vi "test-ramsete-path.vi"() -> ()   [LabVIEW 2019]
uses:
  Pathfinder-Lib/VIs/Waypoint.ctl
  Pathfinder-Lib/VIs/Wheel_Ctrl_Path_Element.ctl
  PathExecution_Library/PATH_SAMPLE.ctl
  PathExecution_Library/POSE.ctl
  PathExecution_Library/TRANSLATION.ctl
  PathExecution_Library/ROTATION.ctl
  Pathfinder-Lib/VIs/Wheel_Ctrl_Path.ctl
  Pathfinder-Lib/Pathfinder.lvlib
  Secret_Control_Library_Protected/Secret_Control_Library_Protected.lvlib
  PathExecution_Library/PathExecution_Library.lvlib
panel:
  in  "Tab Control 3":enum32{"Robot Data", "Path Definition"}(tab)
  in  "Real max\n speed":dbl=96.0
  in  "wheelbase_width":dbl=20.866
  in  "max_jerk":dbl=90.0
  in  "max_acceleration":dbl=65.0
  in  "max_velocity":dbl=72.0
  in  "?":T1[](array[typedef])=[{"x"=15.0, "y"=105.0, "angle"=0.0}, {"x"=35.0, "y"=105.0, "angle"=0.0}, {"x"=210.0, "y"=185.0, "angle"=60.0}]
  in  "Path Results\ndT":dbl=0.02 format="%7.3f"
  in  "sample_count":i32=100000
  out "Path calculation error":errorcluster
  in  "Calculate\nPath":bool
  out "Complete,\nReady to \nExecute":bool
  out "Path \nSpeed > \nMax":bool
  in  "Rev\nDirection":bool
  out "max speed":dbl
  in  "Tab Control 2":T2(tab)
  in  "Enable Ramsete":bool=TRUE
  out "Distance":dbl[](array[numeric]) format="%19.2f"
  in  "Execute\nRobot":bool
  out "Robot\nExecuting":bool
  in  "Stop\nProgram":bool
  out "Speed":dbl[](array[numeric]) format="%19.2f"
  out "SpeedDmd":dbl[](array[numeric]) format="%19.2f"
  in  "Next Step":bool
  in  "Include Step":bool=TRUE
  in  "End Path CMD":i32=64
  in  "Cont Path CMD":i32=62
  in  "Start Path CMD":i32=60
  in  "Starting Step":i32
  in  "Command List Path Comment":string
  in  "Command List File Name":path
  in  "CreateCmdList":bool
  in  "CreateCmdList 2":bool
  in  "Command List File Name 2":path
  in  "Command List Path Comment 2":string
  in  "Starting Step 2":i32
  in  "Start Path CMD 2":i32=80
  in  "Cont Path CMD 2":i32=82
  in  "End Path CMD 2":i32=84
  in  "Include Step 2":bool=TRUE
  in  "Tab Control":T3(tab)
  out "Position":cluster{dbl[], dbl[]}[](graph)
  out "Path":T4(graph)
  out "Size":i32
  out "Robot Path Data":T5[](array[typedef]) {"D Time" format="%13.3f"; "Angle" format="%13.3f"; "R dist" format="%13.3f"; "L dist" format="%13.3f"; "R spd" format="%13.3f"; "L spd" format="%13.3f"; "T Time" format="%13.3f"}
  out "Ramsete Path":T6[](array[typedef])
  out "element":T6
  out "AtReference":bool
  out "size(s)":i32
  out "Path INX":i32
  out "size(s) 2":i32
  out "Err Pose":T7 {"ROTATION"."SIN" format="%10.3f"; "ROTATION"."COS" format="%10.3f"; "ROTATION"."VALUE" format="%10.3f"; "TRANSLATION"."Y" format="%9.3f"; "TRANSLATION"."X" format="%10.3f"}
  out "CurrentRelativePose":T7
  out "Des Pose":T7
  # "ROBOT DATA"
  # "INCHES/SEC"
  # "INCHES/SEC"
  # "INCHES/SEC^2"
  # "?? INCHES/SEC^3"
  # "Simulated robot is 20.866"
  # "INCHES"
  # "PATH DEFINITION"
  # "SEC"
  # "ROBOT EXECUTION"
  # "Instructions:\nThis should create a path, show the data on the various tabs and optionally write the motor demands and expected results to a file for use on a a robot..\n1) Enter robot data on Robot Data Tab\n2) Define your path definitions.\n3) Define the time increment.  0.020 is chosen since that matches the normal loop time.\n4) Press calculate path.  If a good path was calculated it will be displayed on the Tank Data tab, and the Ready to Execute will indicate execution can begin.\nThe path can be recalculated many times before selecting execute.\n\nTo write to a file.\n5) Select the file name\n6) This example uses \"steps\", sequential numbers for inclusion into a list based autonomous routine.  Including the step number if optional.\n7) This uses command numbers to indicate first, last, and intermediate steps.  This allows some simplification of the execution routine.  It\nalso allows the path to be executed backwards if desired.  The command numbers are changeable.\n8) Press \"Create Command List\".\n\nNotes:\n- PC robot simulataion is disabled in this program.  The code is still there if you want to restore it and try it out.  Use one of the other test programs \nto simulate the path on a PC.\n- The path generation logic doesn't account distribution of speed to the left and right wheels.  As a result the maximum speed can be exceeded.\nIf this happens, but Path Speed > Max light will light and Ready to Execute will not light.  Lower the maximum speed in the Robot Data tab\nand recalulate the path.\n- 2019 playing field size - width: 26 ft 11.25 In = 323.25 in , length: 52 ft 5.25 in = 629.25 in  (I didn't verify this for the 2020 version.)"
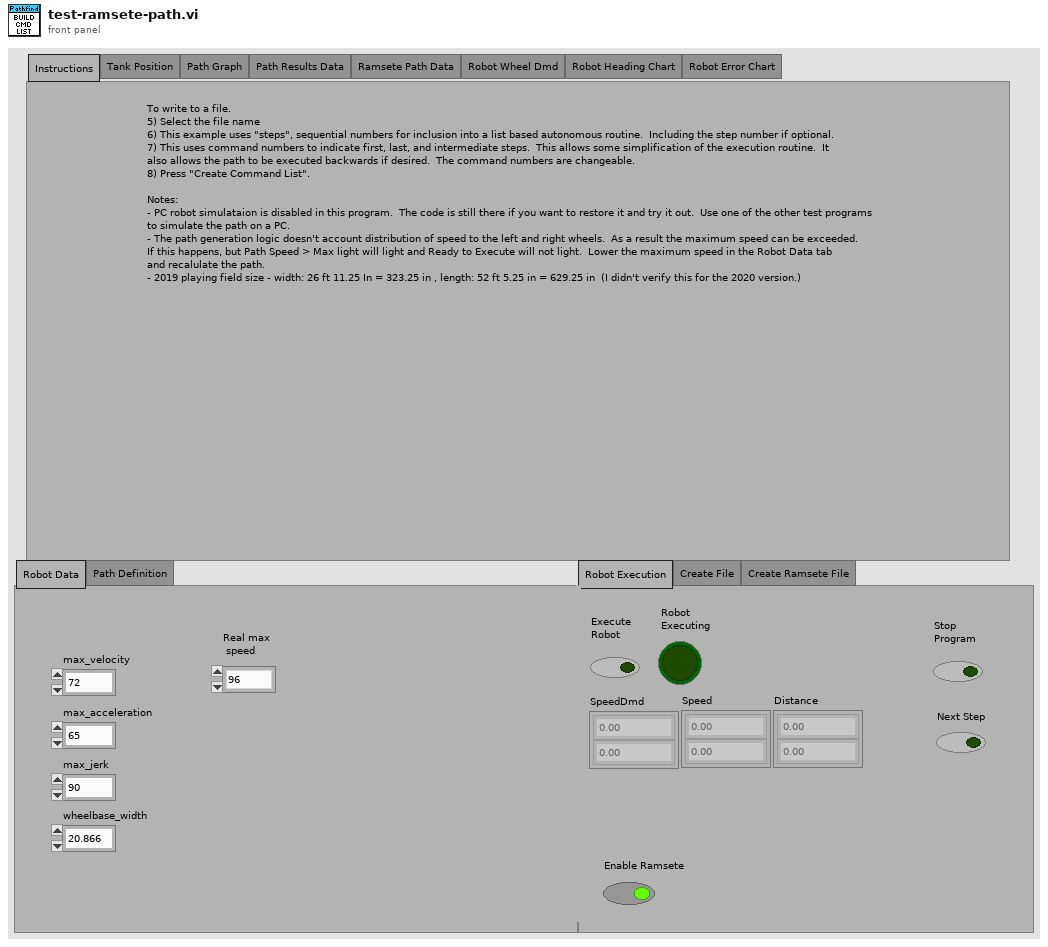
[diagram p1: front panel]
types:
  T1 = typedef "Pathfinder.lvlib/Waypoint.ctl" = cluster{"x":dbl, "y":dbl, "angle":dbl}
  T2 = enum32{"Robot Execution", "Create File", "Create Ramsete File"}
  T3 = enum32{"Instructions", "Tank Position", "Path Graph", "Path Results Data", "Ramsete Path Data", "Robot Wheel Dmd", "Robot Heading Chart", "Robot Error Chart"}
  T4 = cluster{"position":dbl, "velocity":dbl, "acceleration":dbl, "jerk":dbl, "heading":dbl}[]
  T5 = typedef "Pathfinder.lvlib/Wheel_Ctrl_Path_Element.ctl" = cluster{"T Time":dbl, "L spd":dbl, "R spd":dbl, "L dist":dbl, "R dist":dbl, "Angle":dbl, "D Time":dbl}
  T6 = typedef "PathExecution_Library.lvlib/PATH_SAMPLE.ctl" = cluster{"Path Lin Vel":dbl, "Path Ang Vel":dbl, "Path X":dbl, "Path Y":dbl, "Path Heading":dbl, "Path Time Off":dbl}
  T7 = typedef "PathExecution_Library.lvlib/POSE.ctl" = cluster{"TRANSLATION":T8, "ROTATION":T9}
  T8 = typedef "PathExecution_Library.lvlib/TRANSLATION.ctl" = cluster{"X":dbl, "Y":dbl}
  T9 = typedef "PathExecution_Library.lvlib/ROTATION.ctl" = cluster{"VALUE":dbl, "COS":dbl, "SIN":dbl}
  T10 = typedef "Pathfinder.lvlib/Wheel_Ctrl_Path.ctl" = cluster{"Wheel_Ctrl_Elements":T5[], "NumberOfElements":u32, "DeltaMillseconds":i32}
  T11 = typedef "Pathfinder.lvlib/Segment.ctl" = cluster{"dt":dbl, "x":dbl, "y":dbl, "position":dbl, "velocity":dbl, "acceleration":dbl, "jerk":dbl, "heading":dbl}
  T12 = cluster{"position":dbl, "velocity":dbl, "acceleration":dbl, "jerk":dbl, "heading":dbl}
  T13 = typedef "PathExecution_Library.lvlib/CHASSIS.ctl" = cluster{"vX":dbl, "vY":dbl, "vOmega":dbl}
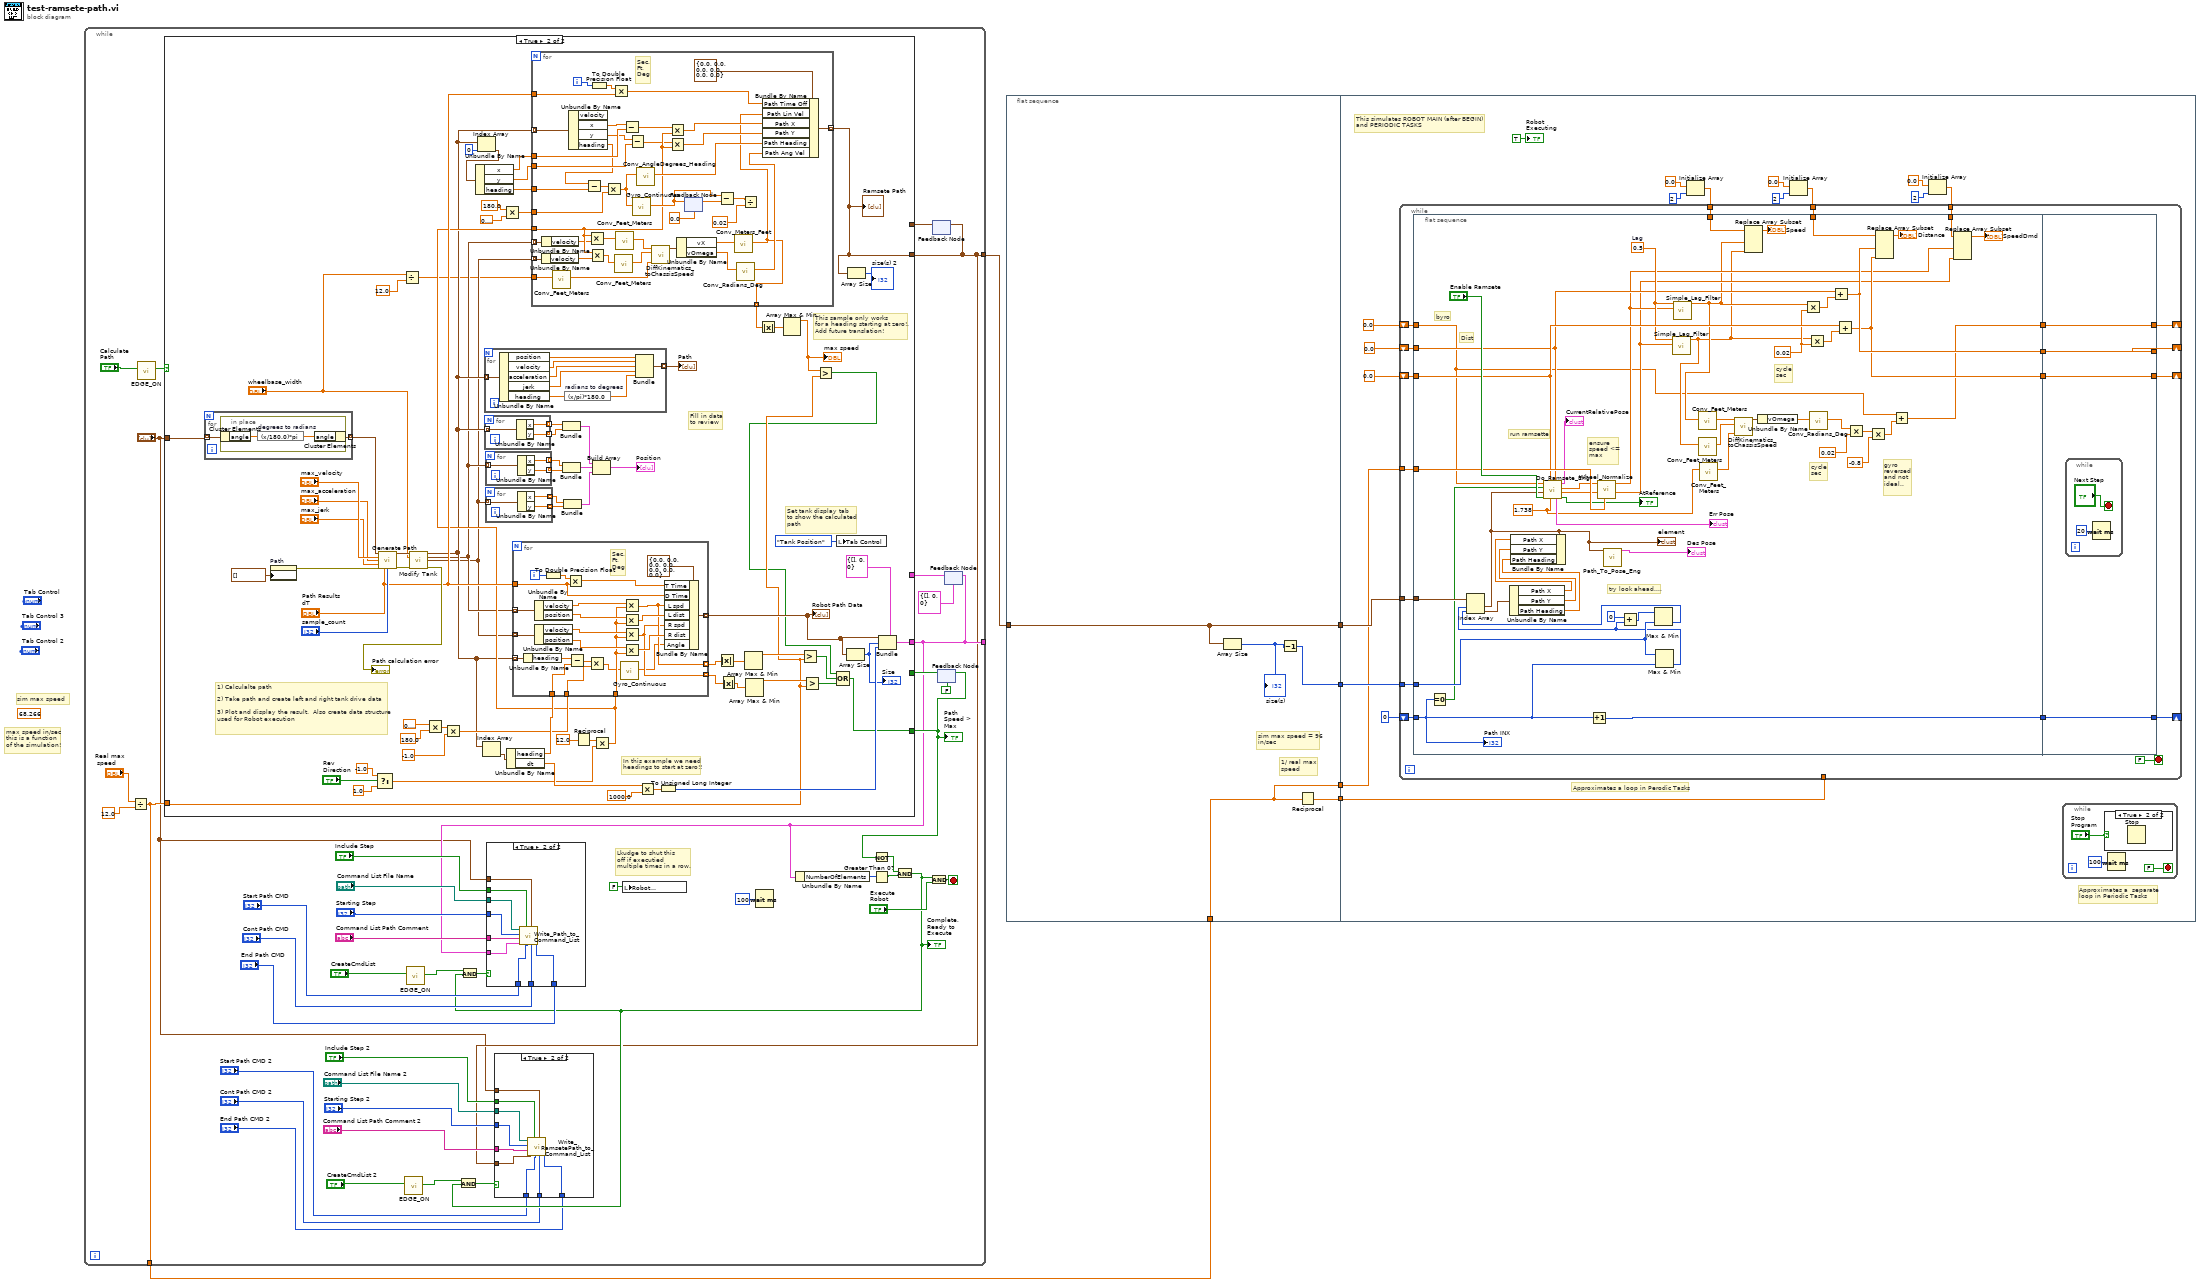
[diagram p0: block diagram]
diagram:
  (unwired) 68.266 ("x")
  # "sim max speed"
  # "max speed in/sec\nthis is a function\nof the simulation!"
  n1 = while {
    tunnel: [w22] -> w6
    tunnel: [w21] -> _
    tunnel: [w8] -> w4
    stop <- w41 stop-if-true
    # "Lkudge to shut this\noff if executied\nmultiple times in a row."
    n2 = Divide(x="Real max\n speed", y=12.0) -> (x/y=w22:dbl)
    n3 = call "EDGE_ON.vi"("INPUT"="Calculate\nPath") -> ("EDGE ON"=w46:bool)  [unwired: 10 in]
    n4 = call "EDGE_ON.vi"("INPUT"="CreateCmdList 2") -> ("EDGE ON"=w15:bool)  [unwired: 10 in]
    n5 = call "EDGE_ON.vi"("INPUT"="CreateCmdList") -> ("EDGE ON"=w29:bool)  [unwired: 10 in]
    n6 = local write "Robot\nExecuting"(FALSE ("Robot\nExecuting")) -> ()
    n7 = Wait (ms)(milliseconds to wait=u32 100) -> ()  [unwired: 1 out]
    n8 = feedback #1() -> (w20:T6[])  [unwired: 1 in]
    n9 = feedback #2(FALSE) -> (w38:bool)
    n10 = feedback #3(T10 {"Wheel_Ctrl_Elements"=[], "NumberOfElements"=0, "DeltaMillseconds"=0} ("Wheel_Ctrl_Elements")) -> (w44:T10)
    n11 = case shown="True" w46 {
      tunnel: [w69 w113] -> w21
      tunnel: w44 -> [w69 _]
      tunnel: w22 -> [_ w72]
      tunnel: [w68 w110] -> w35
      tunnel: w38 -> [w68 _]
      tunnel: "?" -> [_ w108]
      tunnel: [w67 w92] -> w8
      tunnel: w20 -> [w67 _]
      frame False {
      }
      frame True {
        # "This sample only works\nfor a heading starting at zero!.\nAdd future translation!"
        # "Set tank display tab\nto show the calculated\npath"
        # "Fill in data\nto review"
        # "1) Calculalte path\n\n2) Take path and create left and right tank drive data\n\n3) Plot and display the result.  Also create data structure\nused for Robot execution"
        # "In this example we need\nheadings to start at zero!!"
        n12 = for {
          tunnel: w108 -> [w213] mode=indexing
          tunnel: [w212] -> w138 mode=indexing
          n13 = in-place {
            n14 = in-place-cluster #4(w213) -> ("angle"=w215:dbl)
            n15 = expression code="(x/180.0)*pi" "degrees to radians"(w215) -> (w214:dbl)
            n16 = in-place-cluster #4("angle"=w214) -> (w212:T1)
          }
        }
        n17 = property on="Path" class="WFChart (strict)"("History Data"=T4 []) -> (error out=w139:errorcluster)  [unwired: 2 in, 1 out]
        n18 = Select(t=-1.0, s="Rev\nDirection", f=1.0) -> (s? t:f=w103:dbl)
        n19 = call "Generate Path.vi"("path"=w138, "max_velocity"="max_velocity", "max_acceleration"="max_acceleration", "max_jerk"="max_jerk", "error in"=w139, "dt (.001)"="Path Results\ndT", "sample_count (100000)"="sample_count") -> ("Segments"=w140:T11[], "error out"=w128:errorcluster)  [unwired: 7 in]
        n20 = Divide(x="wheelbase_width", y=12.0) -> (x/y=w82:dbl)
        n21 = call "Modify Tank.vi"("Original"=w140, "wheelbase_width"="wheelbase_width", "error in"=w128) -> ("original"=w97:T11[], "left"=w86:T11[], "right"=w85:T11[], "error out"=→"Path calculation error":errorcluster)  [unwired: 9 in]
        n22 = Multiply(x=0.3183098861837907, y=180.0) -> (x*y=w144:dbl)
        n23 = Multiply(x=w144, y=-1.0) -> (x*y=w100:dbl)
        n24 = Index Array(array=w97, index=0) -> (element=w95:T11)
        n25 = Unbundle By Name(w95) -> ("x"=w94:dbl, "y"=w93:dbl, "heading"=w90:dbl)
        n26 = Index Array(array=w97) -> (element=w145:T11)  [unwired: 1 in]
        n27 = for {
          tunnel: w97 -> [w232] mode=indexing
          tunnel: [w226] -> w142 mode=indexing
          n28 = Unbundle By Name(w232) -> ("position"=w231:dbl, "velocity"=w230:dbl, "acceleration"=w229:dbl, "jerk"=w228:dbl, "heading"=w227:dbl)
          n29 = expression code="(x/pi)*180.0" "radians to degrees"(w227) -> (w225:dbl)
          n30 = Bundle("position"=w231, "velocity"=w230, "acceleration"=w229, "jerk"=w228, "heading"=w225) -> (w226:T12)  [unwired: 1 in]
        }
        "Path" <- w142
        n31 = for {
          tunnel: w97 -> [w218] mode=indexing
          tunnel: [w217] -> w135 mode=indexing
          tunnel: [w216] -> w136 mode=indexing
          n32 = Unbundle By Name(w218) -> ("x"=w217:dbl, "y"=w216:dbl)
        }
        n33 = for {
          tunnel: w86 -> [w224] mode=indexing
          tunnel: [w223] -> w129 mode=indexing
          tunnel: [w222] -> w130 mode=indexing
          n34 = Unbundle By Name(w224) -> ("x"=w223:dbl, "y"=w222:dbl)
        }
        n35 = for {
          tunnel: w85 -> [w221] mode=indexing
          tunnel: [w220] -> w131 mode=indexing
          tunnel: [w219] -> w132 mode=indexing
          n36 = Unbundle By Name(w221) -> ("x"=w220:dbl, "y"=w219:dbl)
        }
        n37 = Multiply(x=180.0, y=0.3183098861837907) -> (x*y=w87:dbl)
        n38 = Unbundle By Name(w145) -> ("heading"=w101:dbl, "dt"=w117:dbl)
        n39 = Bundle(w135, w136) -> (w137:cluster{dbl[], dbl[]})  [unwired: 1 in]
        n40 = Bundle(w129, w130) -> (w134:cluster{dbl[], dbl[]})  [unwired: 1 in]
        n41 = Bundle(w131, w132) -> (w133:cluster{dbl[], dbl[]})  [unwired: 1 in]
        n42 = Reciprocal(x=12.0) -> (1/x=w107:dbl)
        n43 = Build Array(w137, w134, w133) -> (→"Position":cluster{dbl[], dbl[]}[])
        n44 = Multiply(x=w107, y=w103) -> (x*y=w99:dbl)
        n45 = for {
          tunnel: "Path Results\ndT" -> [w207]
          tunnel: [w210] -> w109 mode=indexing
          tunnel: w99 -> [w202]
          tunnel: w86 -> [w199] mode=indexing
          tunnel: w85 -> [w198] mode=indexing
          tunnel: w97 -> [w197] mode=indexing
          tunnel: w101 -> [w190]
          tunnel: [w193] -> w81 mode=indexing
          tunnel: [w192] -> w78 mode=indexing
          tunnel: w100 -> [w191]
          i -> [w209]
          # "Sec,\nFt,\nDeg"
          n46 = Unbundle By Name(w197) -> ("heading"=w195:dbl)
          n47 = Unbundle By Name(w199) -> ("velocity"=w206:dbl, "position"=w205:dbl)
          n48 = Unbundle By Name(w198) -> ("velocity"=w204:dbl, "position"=w203:dbl)
          n49 = To Double Precision Float(number=w209) -> (double precision float=w211:dbl)
          n50 = Multiply(x=w211, y=w207) -> (x*y=w208:dbl)
          n51 = Subtract(x=w195, y=w190) -> (x-y=w196:dbl)
          n52 = Multiply(x=w196, y=w191) -> (x*y=w189:dbl)
          n53 = call "Gyro_Continuous.vi"("GyroInput"=w189) -> ("GyroContinuous"=w188:dbl)  [unwired: 10 in]
          n54 = Multiply(x=w206, y=w202) -> (x*y=w193:dbl)
          n55 = Multiply(x=w205, y=w202) -> (x*y=w201:dbl)
          n56 = Multiply(x=w204, y=w202) -> (x*y=w192:dbl)
          n57 = Multiply(x=w203, y=w202) -> (x*y=w200:dbl)
          n58 = Bundle By Name(cluster=T5 {"T Time"=0.0, "L spd"=0.0, "R spd"=0.0, "L dist"=0.0, "R dist"=0.0, "Angle"=0.0, "D Time"=0.0} ("Wheel dmd"), "T Time"=w208, "D Time"=w207, "L spd"=w193, "L dist"=w201, "R spd"=w192, "R dist"=w200, "Angle"=w188) -> (w210:T5)
        }
        "Robot Path Data" <- w109
        n59 = for {
          tunnel: "Path Results\ndT" -> [w185]
          tunnel: w99 -> [w160]
          tunnel: w97 -> [w184] mode=indexing
          tunnel: [w178] -> w92 mode=indexing
          tunnel: w94 -> [w171]
          tunnel: w93 -> [w169]
          tunnel: w90 -> [w166]
          tunnel: w87 -> [w163]
          tunnel: w86 -> [w162] mode=indexing
          tunnel: w85 -> [w161] mode=indexing
          tunnel: w82 -> [w157]
          tunnel: [w147] -> w73 mode=indexing
          i -> [w186]
          # "Sec,\nFt,\nDeg"
          n60 = Unbundle By Name(w161) -> ("velocity"=w158:dbl)
          n61 = Unbundle By Name(w162) -> ("velocity"=w159:dbl)
          n62 = call "Conv_Feet_Meters.vi"("Feet"=w157) -> ("Meters"=w152:dbl)  [unwired: 10 in]
          n63 = Unbundle By Name(w184) -> ("x"=w172:dbl, "y"=w170:dbl, "heading"=w167:dbl)  [unwired: 1 out]
          n64 = Subtract(x=w167, y=w166) -> (x-y=w182:dbl)
          n65 = Multiply(x=w160, y=w159) -> (x*y=w156:dbl)
          n66 = Multiply(x=w160, y=w158) -> (x*y=w155:dbl)
          n67 = To Double Precision Float(number=w186) -> (double precision float=w187:dbl)
          n68 = Multiply(x=w182, y=w163) -> (x*y=w165:dbl)
          n69 = Multiply(x=w187, y=w185) -> (x*y=w181:dbl)
          n70 = call "Conv_Feet_Meters.vi"("Feet"=w155) -> ("Meters"=w153:dbl)  [unwired: 10 in]
          n71 = call "Conv_Feet_Meters.vi"("Feet"=w156) -> ("Meters"=w154:dbl)  [unwired: 10 in]
          n72 = Subtract(x=w172, y=w171) -> (x-y=w168:dbl)
          n73 = Subtract(x=w170, y=w169) -> (x-y=w146:dbl)
          n74 = call "Gyro_Continuous.vi"("GyroInput"=w165) -> ("GyroContinuous"=w173:dbl)  [unwired: 10 in]
          n75 = call "Conv_AngleDegrees_Heading.vi"("Degrees"=w165) -> ("Radians"=w164:dbl)  [unwired: 10 in]
          n76 = call "DiffKinematics_toChassisSpeed.vi"("TrackWidth_Meters"=w152, "RightVelocity"=w153, "LeftVelocity"=w154) -> ("CHASSIS Speed"=w151:T13)  [unwired: 8 in]
          n77 = Multiply(x=w168, y=w160) -> (x*y=w180:dbl)
          n78 = Multiply(x=w146, y=w160) -> (x*y=w179:dbl)
          n79 = Unbundle By Name(w151) -> ("vX"=w150:dbl, "vOmega"=w149:dbl)
          n80 = feedback-in #5(w173) -> ()
          n81 = feedback #5(0.0) -> (w176:dbl)
          n82 = Subtract(x=w173, y=w176) -> (x-y=w175:dbl)
          n83 = call "Conv_Meters_Feet.vi"("Meters"=w150) -> ("Feet"=w147:dbl)  [unwired: 10 in]
          n84 = call "Conv_Radians_Deg.vi"("Radians"=w149) -> ("Degrees"=w148:dbl)  [unwired: 10 in]
          n85 = Divide(x=w175, y=0.02) -> ()  [unwired: 1 out]
          n86 = Bundle By Name(cluster=T6 {"Path Lin Vel"=0.0, "Path Ang Vel"=0.0, "Path X"=0.0, "Path Y"=0.0, "Path Heading"=0.0, "Path Time Off"=0.0} ("Path Sample"), "Path Time Off"=w181, "Path Lin Vel"=w147, "Path X"=w180, "Path Y"=w179, "Path Heading"=w164, "Path Ang Vel"=w148) -> (w178:T6)
        }
        "Ramsete Path" <- w92
        n87 = Multiply(x=w117, y=1000.0) -> (x*y=w115:dbl)
        n88 = To Unsigned Long Integer(number=w115) -> (unsigned 32bit integer=w114:u32)
        n89 = Absolute Value(x=w81) -> (abs(x)=w80:dbl[])
        n90 = Absolute Value(x=w78) -> (abs(x)=w76:dbl[])
        n91 = Array Max & Min(array=w80) -> (max value=w79:dbl)  [unwired: 3 out]
        n92 = Array Max & Min(array=w76) -> (max value=w77:dbl)  [unwired: 3 out]
        n93 = Absolute Value(x=w73) -> (abs(x)=w74:dbl[])
        n94 = Array Max & Min(array=w74) -> (max value=w71:dbl)  [unwired: 3 out]
        "max speed" <- w71
        n95 = Greater?(x=w79, y=w72) -> (0:w111:bool)
        n96 = Greater?(x=w77, y=w72) -> (0:w75:bool)
        n97 = Greater?(x=w71, y=w72) -> (0:w70:bool)
        n98 = Compound Arithmetic op=OR(w70, w111, w75) -> (w110:bool)
        n99 = local write "Tab Control"(T3."Tank Position" ("Tab Control")) -> ()
        n100 = Array Size(array=w109) -> (size(s)=w112:i32)
        "Size" <- w112
        n101 = Array Size(array=w92) -> (size(s)=→"size(s) 2":i32)
        n102 = Bundle(cluster=T10 {"Wheel_Ctrl_Elements"=[], "NumberOfElements"=0, "DeltaMillseconds"=0} ("Wheel_Ctrl_Elements"), "Wheel_Ctrl_Elements"=w109, "NumberOfElements"=w112, "DeltaMillseconds"=w114) -> (w113:T10)
      }
    }
    "Path \nSpeed > \nMax" <- w35
    n103 = Unbundle By Name(w21) -> ("NumberOfElements"=w43:u32)
    n104 = Not(x=w35) -> (.not. x?=w36:bool)
    n105 = Greater Than 0?(x=w43) -> (x > 0?=w37:bool)
    n106 = And(x=w36, y=w37) -> (x .and. y?=w13:bool)
    "Complete,\nReady to \nExecute" <- w13
    n107 = And(x=w15, y=w13) -> (x .and. y?=w14:bool)
    n108 = And(x=w29, y=w13) -> (x .and. y?=w30:bool)
    n109 = case shown="True" w30 {
      tunnel: "Command List File Name" -> [_ w66]
      tunnel: "Starting Step" -> [_ w65]
      tunnel: "Command List Path Comment" -> [_ w64]
      tunnel: w21 -> [_ w63]
      tunnel: "End Path CMD" -> [_ w62]
      tunnel: "Cont Path CMD" -> [_ w61]
      tunnel: "Start Path CMD" -> [_ w60]
      tunnel: "Include Step" -> [_ w59]
      tunnel: "?" -> [_ w58]
      frame False {
      }
      frame True {
        n110 = call "Write_Path_to_Command_List.vi"("LastCmdNumb"=w62, "CmdNumb"=w61, "WayPoints"=w58, "FirstCmdNumb"=w60, "Include Step"=w59, "Wheel_Ctrl_Elements"=w63, "Comment"=w64, "starting step"=w65, "Cmd List File"=w66) -> ()  [unwired: 3 in]
      }
    }
    n111 = case shown="True" w14 {
      tunnel: "Command List File Name 2" -> [_ w57]
      tunnel: "Starting Step 2" -> [_ w56]
      tunnel: "Command List Path Comment 2" -> [_ w55]
      tunnel: w8 -> [_ w49]
      tunnel: "End Path CMD 2" -> [_ w54]
      tunnel: "Cont Path CMD 2" -> [_ w53]
      tunnel: "Start Path CMD 2" -> [_ w52]
      tunnel: "Include Step 2" -> [_ w51]
      tunnel: "?" -> [_ w50]
      frame False {
      }
      frame True {
        n112 = call "Write_RamsetePath_to_Command_List.vi"("LastCmdNumb"=w54, "CmdNumb"=w53, "WayPoints"=w50, "FirstCmdNumb"=w52, "Include Step"=w51, "Path Sample Array"=w49, "Comment"=w55, "starting step"=w56, "Cmd List File"=w57) -> ()  [unwired: 3 in]
      }
    }
    n113 = And(x=w13, y="Execute\nRobot") -> (x .and. y?=w41:bool)
    n114 = feedback-in #1(w8) -> ()
    n115 = feedback-in #2(w35) -> ()
    n116 = feedback-in #3(w21) -> ()
  }
  n117 = flat-sequence {
    tunnel: [w237] -> w5
    tunnel: w6 -> [w233]
    tunnel: w4 -> [w236]
    tunnel: [w236] -> w3
    tunnel: [w234] -> w2
    tunnel: [w233] -> w1
    tunnel: w5 -> [w247]
    tunnel: w3 -> [w252]
    tunnel: w2 -> [w251]
    tunnel: w1 -> [w242]
    frame #0 {
      # "sim max speed = 96\nin/sec"
      # "1/ real max \nspeed"
      n118 = Array Size(array=w236) -> (size(s)=w235:i32)
      "size(s)" <- w235
      n119 = Decrement(x=w235) -> (x-1=w234:i32)
      n120 = Reciprocal(x=w233) -> (1/x=w237:dbl)
    }
    frame #1 {
      # "Approximates a  separate\nloop in Periodic Tasks"
      # "This simulates ROBOT MAIN (after BEGIN)\nand PERIODIC TASKS"
      # "Approximates a loop in Perodic Tasks"
      n121 = Initialize Array(0.0, 2 ("dimension size")) -> (w244:dbl[])
      n122 = Initialize Array(0.0, 2 ("dimension size")) -> (w248:dbl[])
      n123 = Initialize Array(0.0, 2 ("dimension size")) -> (w243:dbl[])
      n124 = while {
        shift-right: [w277] -> _
        shift-left: 0 -> [w273]
        tunnel: w244 -> [w271]
        tunnel: w252 -> [w275]
        tunnel: w251 -> [w274]
        tunnel: w248 -> [w272]
        tunnel: w247 -> [_]
        tunnel: w243 -> [w270]
        tunnel: w242 -> [w269]
        shift-right: [w268] -> _
        shift-left: 0.0 -> [w264]
        shift-right: [w267] -> _
        shift-left: 0.0 -> [w266]
        shift-right: [w265] -> _
        shift-left: 0.0 -> [w263]
        stop <- FALSE stop-if-true
        n125 = flat-sequence {
          tunnel: w275 -> [w327]
          tunnel: w274 -> [w326]
          tunnel: w273 -> [w325]
          tunnel: w272 -> [w323]
          tunnel: w271 -> [w322]
          tunnel: w270 -> [w320]
          tunnel: w269 -> [w319]
          tunnel: w266 -> [w314]
          tunnel: w264 -> [w296]
          tunnel: w263 -> [w281]
          tunnel: [w330] -> w262
          tunnel: [w316] -> w261
          tunnel: [w315] -> w260
          tunnel: [w282] -> w259
          tunnel: [w331] -> w265
          tunnel: [w332] -> w267
          tunnel: [w333] -> w268
          tunnel: [w334] -> w277
          tunnel: w262 -> [w334]
          tunnel: w261 -> [w333]
          tunnel: w260 -> [w332]
          tunnel: w259 -> [w331]
          frame #0 {
            w292 = 1.738 ("WheelBase-Feet")
            w295 = 0.02 ("y")
            w297 = 0.5  # Lag
            # "cycle\nsec"
            # "cycle\nsec"
            # "gyro\nreversed\nand not\nideal.."
            # "byro"
            # "ensure \nspeed <=\nmax"
            # "try look ahead...."
            # "run ramsette"
            # "Dist"
            n126 = Equal To 0?(x=w325) -> (x = 0?=w304:bool)
            n127 = Increment(x=w325) -> (x+1=w330:i32)
            n128 = Max & Min(x=w326, y=w325) -> (min(x,y)=w305:i32)  [unwired: 1 out]
            n129 = Add(x=0, y=w305) -> (x+y=w307:i32)
            n130 = Max & Min(x=w307, y=w326) -> (min(x,y)=w306:i32)  [unwired: 1 out]
            n131 = Index Array(array=w327, index #1=w305, index #2=w306) -> (element #1=w299:T6, element #2=w303:T6)
            "element" <- w299
            n132 = Unbundle By Name(w303) -> ("Path X"=w302:dbl, "Path Y"=w301:dbl, "Path Heading"=w300:dbl)
            n133 = Bundle By Name(cluster=w299, "Path X"=w302, "Path Y"=w301, "Path Heading"=w300) -> ()  [unwired: 1 out]
            n134 = call "Do_Ramsete_Eng.vi"("LeftDist-Feet"=w296, "WheelBase-Feet"=w292, "RightDist-Feet"=w314, "Ramsete Enable"="Enable Ramsete", "Path Sample"=w299, "Reset"=w304, "Gyro-Deg"=w281) -> ("AtReference"=→"AtReference":bool, "RightVelDmd"=w309:dbl, "LeftVelDmd"=w310:dbl, "CurrentRelativePose"=→"CurrentRelativePose":T7, "Err Pose"=→"Err Pose":T7)
            n135 = call "Wheel_Normalize.vi"("Max Speed"=w319, "Right Wheel Demand"=w309, "Left Wheel Demand"=w310) -> ("Normalized Right Wheel Demand"=w289:dbl, "Normalized Left Wheel Demand"=w290:dbl)  [unwired: 7 in]
            n136 = call "Path_To_Pose_Eng.vi"("Path Sample"=w299) -> ("out POSe"=→"Des Pose":T7)  [unwired: 10 in]
            n137 = call "Simple_Lag_Filter.vi"("Input"=w289, "Lag"=w297) -> ("Lagged Ouptut"=w285:dbl)  [unwired: 9 in]
            n138 = call "Simple_Lag_Filter.vi"("Input"=w290, "Lag"=w297) -> ("Lagged Ouptut"=w286:dbl)  [unwired: 9 in]
            n139 = call "Conv_Feet_Meters.vi"("Feet"=w286) -> ("Meters"=w294:dbl)  [unwired: 10 in]
            n140 = call "Conv_Feet_Meters.vi"("Feet"=w285) -> ("Meters"=w293:dbl)  [unwired: 10 in]
            n141 = call "Conv_Feet_Meters.vi"("Feet"=w292) -> ("Meters"=w291:dbl)  [unwired: 10 in]
            n142 = call "DiffKinematics_toChassisSpeed.vi"("TrackWidth_Meters"=w291, "RightVelocity"=w293, "LeftVelocity"=w294) -> ("CHASSIS Speed"=w288:T13)  [unwired: 8 in]
            n143 = Replace Array Subset(array=w322, new element #1=w286, new element #2=w285) -> (→"Speed":dbl[])  [unwired: 2 in]
            n144 = Unbundle By Name(w288) -> ("vOmega"=w287:dbl)
            n145 = Multiply(x=w286, y=w295) -> (x*y=w318:dbl)
            n146 = Multiply(x=w285, y=w295) -> (x*y=w317:dbl)
            n147 = call "Conv_Radians_Deg.vi"("Radians"=w287) -> ("Degrees"=w283:dbl)  [unwired: 10 in]
            n148 = Add(x=w296, y=w318) -> (x+y=w316:dbl)
            n149 = Add(x=w314, y=w317) -> (x+y=w315:dbl)
            n150 = Multiply(x=w283, y=0.02) -> (x*y=w279:dbl)
            n151 = Multiply(x=w279, y=-0.8 ("x")) -> (x*y=w280:dbl)
            n152 = Replace Array Subset(array=w323, new element #1=w316, new element #2=w315) -> (→"Distance":dbl[])  [unwired: 2 in]
            n153 = Add(x=w281, y=w280) -> (x+y=w282:dbl)
            n154 = Replace Array Subset(array=w320, new element #1=w290, new element #2=w289) -> (→"SpeedDmd":dbl[])  [unwired: 2 in]
            "Path INX" <- w325
          }
          frame #1 {
            n155 = while {
              stop <- "Next Step" stop-if-true
              n156 = Wait (ms)(milliseconds to wait=u32 20) -> ()  [unwired: 1 out]
            }
          }
        }
      }
      n157 = while {
        stop <- FALSE stop-if-true
        n158 = case shown="True" "Stop\nProgram" {
          frame False {
          }
          frame True {
            n159 = Stop() -> ()  [unwired: 1 in]
          }
        }
        n160 = Wait (ms)(milliseconds to wait=u32 100) -> ()  [unwired: 1 out]
      }
      "Robot\nExecuting" <- TRUE ("Robot\nExecuting")
    }
  }
